vi "test_libssh2_channel_window_write_ex.vi"() -> ()   [LabVIEW 2017, in "integration_tests.lvlib"]
uses:
  integration_tests.lvlib
  libssh2/libssh2_channel_open_ex.vi
  libssh2/libssh2_channel_process_startup.vi
  support/support.lvlib
  libssh2/libssh2.lvlib
  <vilib>/PNR/Transparent Assertions/Transparent Assertions/Transparent Assertions.lvlib
panel:
  out "error out":errorcluster
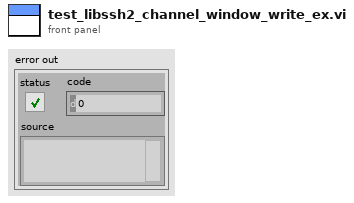
[diagram p1: front panel]
types:
  T1 = typedef "libssh2.lvlib/Session Refnum.ctl" = refnum<k1>
  T2 = typedef "libssh2.lvlib/Channel Refnum.ctl" = refnum<k1>
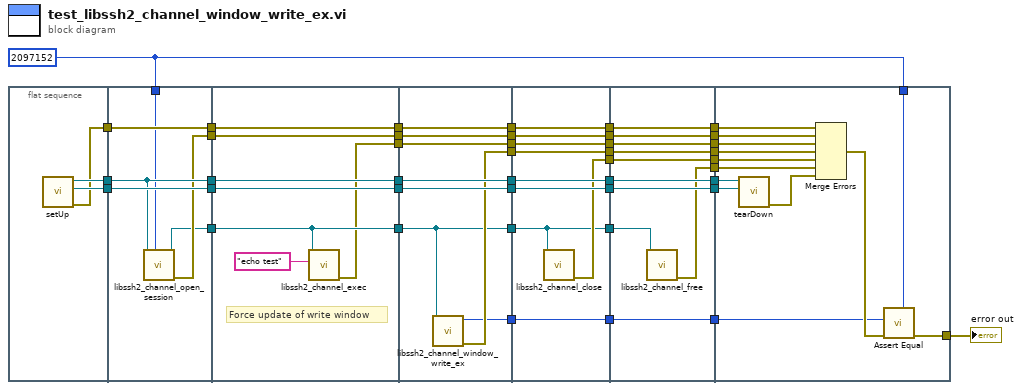
[diagram p0: block diagram]
diagram:
  w23 = u32 2097152 ("window_size (2 MiB)")
  n1 = flat-sequence {
    tunnel: [w45] -> w42
    tunnel: [w44] -> w41
    tunnel: [w43] -> w40
    tunnel: w42 -> [w50]
    tunnel: w41 -> [w51]
    tunnel: [w50] -> w14
    tunnel: [w51] -> w12
    tunnel: w40 -> [w49]
    tunnel: [w49] -> w10
    tunnel: [w48] -> w8
    tunnel: w23 -> [w47]
    tunnel: [w46] -> w6
    tunnel: w14 -> [w58]
    tunnel: [w58] -> w13
    tunnel: w12 -> [w57]
    tunnel: [w57] -> w11
    tunnel: w10 -> [w56]
    tunnel: [w56] -> w9
    tunnel: w8 -> [w55]
    tunnel: [w55] -> w7
    tunnel: w6 -> [w53]
    tunnel: [w53] -> w5
    tunnel: [w52] -> w4
    tunnel: w13 -> [w66]
    tunnel: [w66] -> w21
    tunnel: w11 -> [w65]
    tunnel: [w65] -> w20
    tunnel: w9 -> [w64]
    tunnel: [w64] -> w19
    tunnel: w7 -> [w63]
    tunnel: [w63] -> w18
    tunnel: [w62] -> w17
    tunnel: [w61] -> w16
    tunnel: w5 -> [w60]
    tunnel: [w60] -> w15
    tunnel: w4 -> [w59]
    tunnel: [w59] -> w3
    tunnel: w21 -> [w75]
    tunnel: w20 -> [w74]
    tunnel: [w75] -> w39
    tunnel: [w74] -> w38
    tunnel: [w69] -> w37
    tunnel: [w68] -> w36
    tunnel: [w73] -> w35
    tunnel: w19 -> [w72]
    tunnel: [w72] -> w34
    tunnel: w18 -> [w71]
    tunnel: [w71] -> w33
    tunnel: w17 -> [w70]
    tunnel: [w70] -> w32
    tunnel: w16 -> [w69]
    tunnel: w15 -> [w68]
    tunnel: w3 -> [w67]
    tunnel: [w67] -> w2
    tunnel: w39 -> [w85]
    tunnel: w38 -> [w84]
    tunnel: w37 -> [w83]
    tunnel: w36 -> [w82]
    tunnel: [w85] -> w31
    tunnel: [w84] -> w30
    tunnel: [w83] -> w29
    tunnel: [w81] -> w28
    tunnel: w35 -> [w80]
    tunnel: [w80] -> w27
    tunnel: w34 -> [w79]
    tunnel: [w79] -> w26
    tunnel: w33 -> [w78]
    tunnel: [w78] -> w25
    tunnel: w32 -> [w77]
    tunnel: [w77] -> w24
    tunnel: w2 -> [w76]
    tunnel: [w76] -> w1
    tunnel: w31 -> [w98]
    tunnel: w30 -> [w97]
    tunnel: w29 -> [w88]
    tunnel: [w96] -> w22
    tunnel: w28 -> [w94]
    tunnel: w27 -> [w93]
    tunnel: w26 -> [w92]
    tunnel: w25 -> [w90]
    tunnel: w24 -> [w89]
    tunnel: w23 -> [w87]
    tunnel: w1 -> [w86]
    frame #0 {
      n2 = call "setUp.vi"() -> ("error out"=w43:errorcluster, "connection ID"=w44:refnum<k5>, "session"=w45:T1)  [unwired: 9 in]
    }
    frame #1 {
      n3 = call "libssh2_channel_open_session.vi"("window_size (2 MiB)"=w47, "session"=w50) -> ("error out"=w48:errorcluster, "channel"=w46:T2)  [unwired: 8 in]
    }
    frame #2 {
      # "Force update of write window"
      n4 = call "libssh2_channel_exec.vi"("command"="echo test", "channel"=w53) -> ("error out"=w52:errorcluster)  [unwired: 9 in]
    }
    frame #3 {
      n5 = call "libssh2_channel_window_write_ex.vi"("channel"=w60) -> ("error out"=w62:errorcluster, "remaining write window"=w61:u32)  [unwired: 8 in, 1 out]
    }
    frame #4 {
      n6 = call "libssh2_channel_close.vi"("channel"=w68) -> ("error out"=w73:errorcluster)  [unwired: 10 in]
    }
    frame #5 {
      n7 = call "libssh2_channel_free.vi"("channel"=w82) -> ("error out"=w81:errorcluster)  [unwired: 10 in]
    }
    frame #6 {
      n8 = call "tearDown.vi"("connection ID"=w97, "session"=w98) -> ("error out"=w95:errorcluster)  [unwired: 9 in]
      n9 = Merge Errors(w92, w90, w86, w89, w93, w94, w95) -> (w91:errorcluster)
      n10 = call <vilib>:"Assert Equal.vi"("Expected"=w87, "error in (no error)"=w91, "Actual"=w88) -> ("error out"=w96:errorcluster)  [unwired: 8 in]
    }
  }
  "error out" <- w22
